vi "Set Content Length.vi"(8 "error in (no error)":errorcluster, 11 "Response in":refnum<class "Response.lvclass">) -> (0 "error out":errorcluster, 3 "Response out":refnum<class "Response.lvclass">)   [LabVIEW 2023, in "Response.lvclass"]
uses:
  Response.lvclass
  Response.lvclass/Response.ctl
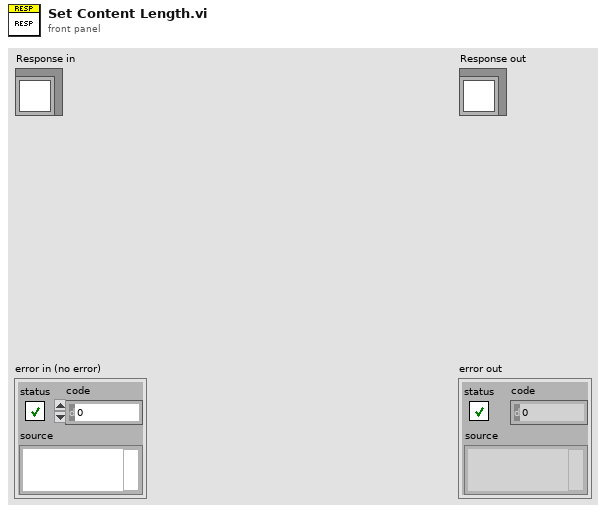
[diagram p1: front panel]
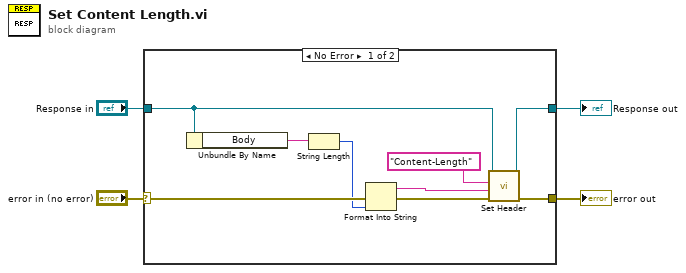
[diagram p0: block diagram]
diagram:
  n1 = case shown="No Error" "error in (no error)" {
    selector: "error in (no error)" -> [w13 w15]
    tunnel: [w12 w15] -> w3
    tunnel: [w11 w14] -> w1
    tunnel: "Response in" -> [w6 w14]
    frame No Error {
      n2 = Unbundle By Name(w6) -> ("Body"=w5:string)
      n3 = String Length(string=w5) -> (length=w8:i32)
      n4 = Format Into String(error in=w13, w8) -> (resulting string=w7:string, error out=w9:errorcluster)  [unwired: 2 in]
      n5 = call "Set Header.vi"("error in (no error)"=w9, "Value"=w7, "Header"="Content-Length", "Response in"=w6) -> ("error out"=w12:errorcluster, "Response out"=w11:refnum<class "Response.lvclass">)  [unwired: 5 in, 1 out]
    }
    frame Error {
    }
  }
  "error out" <- w3
  "Response out" <- w1
